vi "climbingChild.vi"() -> ()   [LabVIEW 2014]
panel:
  out "solutions":i32[][](array[numeric])
  in  "steps":i32=5
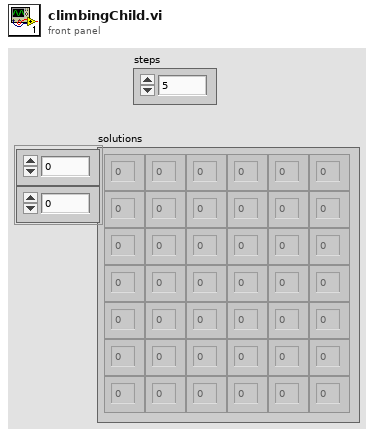
[diagram p1: front panel]
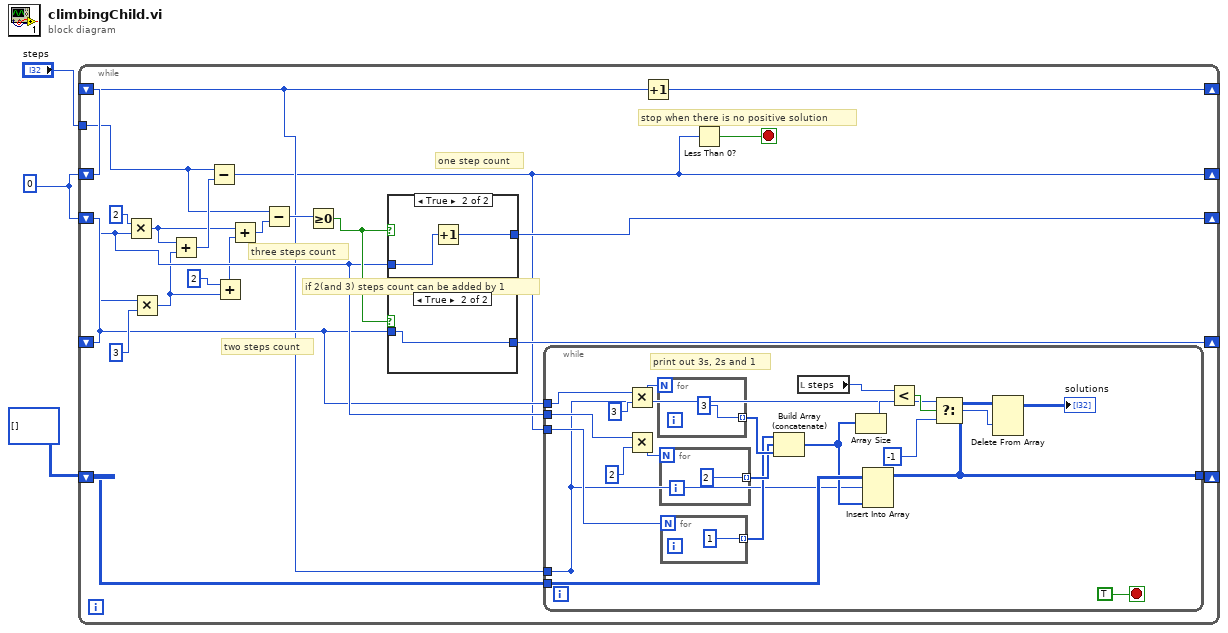
[diagram p0: block diagram]
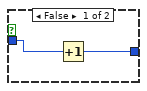
[diagram p2: hidden frame]
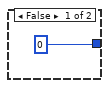
[diagram p3: hidden frame]
diagram:
  w2 = 0
  n1 = while {
    shift-right: [w16] -> _
    shift-left: w2 -> [w15]
    shift-right: [w17] -> _
    shift-left: w2 -> [w14]
    tunnel: "steps" -> [w9]
    shift-right: [w7] -> _
    shift-left: w2 -> [_]
    shift-right: [w12] -> _
    shift-left: w2 -> [w13]
    shift-right: [w11] -> _
    shift-left: i32[][] [] -> [w10]
    stop <- w8 stop-if-true
    # "stop when there is no positive solution"
    # "if 2(and 3) steps count can be added by 1"
    # "three steps count"
    # "two steps count"
    # "one step count"
    n2 = Multiply(x=2, y=w15) -> (x*y=w21:i32)
    n3 = Multiply(x=w14, y=3) -> (x*y=w6:i32)
    n4 = Add(x=w21, y=w6) -> (x+y=w24:i32)
    n5 = Subtract(x=w9, y=w24) -> (x-y=w7:i32)
    n6 = Add(x=2, y=w6) -> (x+y=w5:i32)
    n7 = Add(x=w21, y=w5) -> (x+y=w20:i32)
    n8 = Subtract(x=w9, y=w20) -> (x-y=w19:i32)
    n9 = Greater Or Equal To 0?(x=w19) -> (x >= 0?=w18:bool)
    n10 = case shown="True" w18 {
      tunnel: w15 -> [_ w54]
      tunnel: [0 w53] -> w16
      frame False {
      }
      frame True {
        n11 = Increment(x=w54) -> (x+1=w53:i32)
      }
    }
    n12 = case shown="True" w18 {
      tunnel: w14 -> [w50 w51]
      tunnel: [w49 w51] -> w17
      frame False {
        n13 = Increment(x=w50) -> (x+1=w49:i32)
      }
      frame True {
      }
    }
    n14 = while {
      tunnel: w14 -> [w40]
      tunnel: w15 -> [w44]
      tunnel: w7 -> [w35]
      tunnel: [w26] -> _
      tunnel: w13 -> [w26]
      tunnel: [w33] -> w11
      tunnel: w10 -> [w34]
      stop <- TRUE stop-if-true
      # "print out 3s, 2s and 1"
      n15 = Multiply(x=w40, y=3) -> (x*y=w39:i32)
      n16 = Multiply(x=w44, y=2) -> (x*y=w42:i32)
      n17 = for {
        N: w39 -> [_]
        tunnel: [3] -> w38 mode=indexing
      }
      n18 = for {
        N: w42 -> [_]
        tunnel: [2] -> w37 mode=indexing
      }
      n19 = for {
        N: w35 -> [_]
        tunnel: [1] -> w36 mode=indexing
      }
      n20 = Build Array (concatenate)(w36, w37, w38) -> (w31:i32[])
      n21 = local read "steps"() -> (w29:i32)
      n22 = Array Size(array=w31) -> (size(s)=w30:i32)
      n23 = Insert Into Array(array=w34, index (row)=w26, new element=w31) -> (w33:i32[][])  [unwired: 1 in]
      n24 = Less?(x=w29, y=w30) -> (x < y?=w28:bool)
      n25 = Select(t=w26, s=w28, f=-1) -> (s? t:f=w27:i32)
      n26 = Delete From Array(array=w33, index (row)=w27) -> (array with subset deleted=→"solutions":i32[][])  [unwired: 2 in, 1 out]
    }
    n27 = Increment(x=w13) -> (x+1=w12:i32)
    n28 = Less Than 0?(x=w7) -> (x < 0?=w8:bool)
  }
